vi "Add DataColumn to DataTable.vi"(8 "错误输入（无错误）":errorcluster, 10 "DataColumn":refnum<k24>, 11 "DataTable":refnum<k24>) -> (0 "错误输出":errorcluster, 3 "DataTable":refnum<k24>)   [LabVIEW 2012, in "DataGridView.lvlib"]
uses:
  DataGridView.lvlib
  System.Data
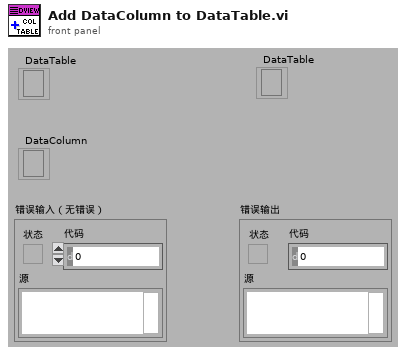
[diagram p1: front panel]
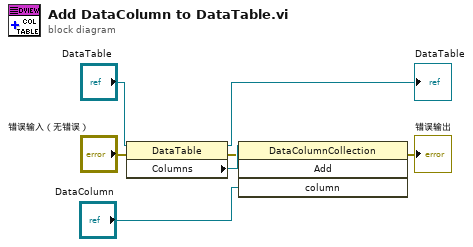
[diagram p0: block diagram]
diagram:
  n1 = property class="DataTable"(reference="DataTable", error in="错误输入（无错误）") -> (reference out=→"DataTable":refnum<k24>, error out=w4:errorcluster, "Columns"=w5:refnum<k24>)
  n2 = invoke class="DataColumnCollection" method="Add"(reference=w5, error in=w4, "column"="DataColumn") -> (error out=→"错误输出":errorcluster)  [unwired: 1 in, 3 out]
